vi "Actor Core.vi"(8 "error in":errorcluster, 11 "Freezer in":refnum<class "Freezer.lvclass">) -> (0 "error out":errorcluster, 3 "Actor out":refnum<class "Actor.lvclass">)   [LabVIEW 2015, in "cRIO-Carbondioxide.lvlib" / "CO2-Actor.lvlib" / "Freezer.lvclass"]
doc: "(<B>Filename</B>: Actor Framework.lvlib:Actor.lvclass:Actor Core.vi)\n\nReceives messages to the actor, reacts to them, and initiates any error handling that may shut the actor down.\n\nDescendant classes may override this VI to append parallel tasks for the actor to complete while it handles messages. Overrides use the Call Parent Method node."
uses:
  Freezer.lvclass
  <vilib>/ActorFramework/Actor/Actor.lvclass
  Freezer.lvclass/Freezer.ctl
  <vilib>/ActorFramework/Actor/Actor.lvclass/Actor.ctl
  <vilib>/ActorFramework/Message Enqueuer/Message Enqueuer.lvclass/Message Enqueuer.ctl
  Freezer Messages/Set Valve Msg/Set Valve Msg.lvclass/Set Valve Msg.ctl
  <vilib>/ActorFramework/Message Enqueuer/Enqueue.vi
  <vilib>/ActorFramework/Actor/Read Self Enqueuer.vi
  <vilib>/ActorFramework/Message Enqueuer/Init from Existing Queue.vi
  <vilib>/ActorFramework/Message Priority Queue/Priority Enqueue.vi
  CO2 Actor/CO2 Actor.lvclass
  Freezer Messages/Set Valve Msg/Set Valve Msg.lvclass
  <vilib>/ActorFramework/Message Enqueuer/Message Enqueuer.lvclass
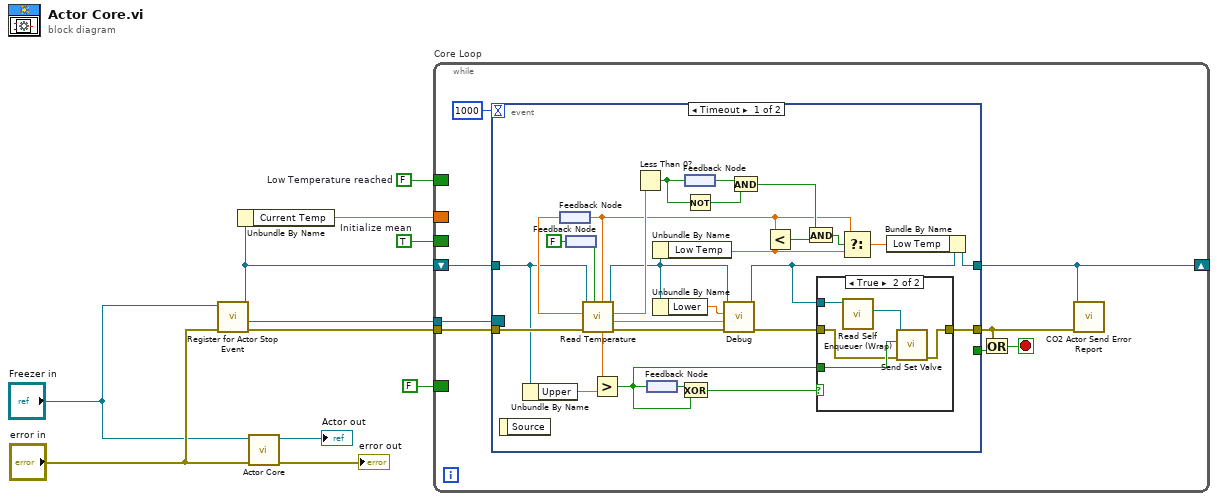
[diagram p0: block diagram]
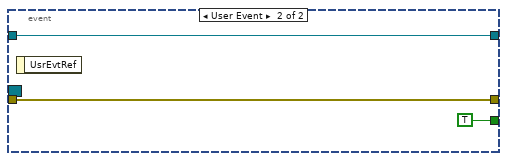
[diagram p3: hidden frame]
diagram:
  w9 = TRUE  # Initialize mean
  w10 = FALSE  # Low Temperature reached
  n1 = call "Register for Actor Stop Event.vi"("error in (no error)"="error in", "CO2 Actor in"="Freezer in") -> ("error out"=w4:errorcluster, "Event Registration Refnum"=w5:refnum<event-registration>, "CO2 Actor out"=w3:refnum<class "Freezer.lvclass">)  [unwired: 7 in]
  n2 = Unbundle By Name(w3) -> ("Current Temp"=w8:dbl)
  n3 = call-parent "Actor Core.vi"("error in"="error in", "CO2 Actor in"="Freezer in") -> ("error out"=→"error out":errorcluster, "Actor out"=→"Actor out":refnum<class "Actor.lvclass">)  [unwired: 8 in]
  n4 = while "Core Loop" {
    tunnel: w4 -> [w19]
    tunnel: w5 -> [w18]
    border: w10 -> [_]
    border: w9 -> [_]
    border: w8 -> [_]
    shift-right: [w12] -> _
    shift-left: w3 -> [w15]
    border: FALSE -> [_]
    stop <- w14 stop-if-true
    n5 = event shown="[0] Timeout" {
      selector: w18 -> [_ _]
      dyn-events: _ -> [_ _]
      timeout: 1000 -> [_ _]
      tunnel: w19 -> [w44 w54]
      tunnel: [_ TRUE] -> w17
      tunnel: w15 -> [w32 w55]
      tunnel: [w33 w54] -> w13
      tunnel: [w39 w55] -> w12
      event Timeout {
        n6 = event-data() -> ()  [unwired: 1 in, 1 out]
        n7 = Unbundle By Name(w32) -> ("Upper"=w31:dbl)
        n8 = feedback #1() -> (w42:dbl)
        n9 = feedback-in #2(FALSE) -> ()
        n10 = feedback #2() -> (w41:bool)
        n11 = call "Read Temperature.vi"("Initialize"=w41, "error in (no error)"=w44, "Current Temperature"=w42, "Freezer in"=w32) -> ("error out"=w25:errorcluster, "dT/dt"=w20:dbl, "dT/dt - Lower"=w40:dbl, "Freezer out"=w23:refnum<class "Freezer.lvclass">, "T - Low Temp"=w37:dbl, "T"=w26:dbl)  [unwired: 2 in]
        n12 = feedback-in #1(w26) -> ()
        n13 = Greater?(x=w37, y=w31) -> (0:w34:bool)
        n14 = Less Than 0?(x=w40) -> (x < 0?=w46:bool)
        n15 = feedback-in #3(w34) -> ()
        n16 = feedback #3() -> (w36:bool)
        n17 = Unbundle By Name(w23) -> ("Low Temp"=w27:dbl)
        n18 = Unbundle By Name(w23) -> ("Lower"=w21:dbl)
        n19 = Exclusive Or(1:w34, 2:w36) -> (0:w35:bool)
        n20 = feedback-in #4(w46) -> ()
        n21 = feedback #4() -> (w47:bool)
        n22 = Not(x=w46) -> (.not. x?=w45:bool)
        n23 = call "Debug.vi"("error in (no error)"=w25, "Numeric 2"=w20, "Numeric 1"=w21, "Freezer in"=w23) -> ("error out"=w24:errorcluster, "Freezer out"=w22:refnum<class "Freezer.lvclass">)  [unwired: 6 in]
        n24 = And(x=w47, y=w45) -> (x .and. y?=w29:bool)
        n25 = Less?(x=w26, y=w27) -> (x < y?=w28:bool)
        n26 = And(x=w29, y=w28) -> (x .and. y?=w30:bool)
        n27 = case shown="True" w35 {
          tunnel: w24 -> [w48 w50]
          tunnel: w22 -> [_ w51]
          tunnel: w34 -> [_ w52]
          tunnel: [w48 w53] -> w33
          frame False {
          }
          frame True {
            n28 = call "Read Self Enqueuer (Wrap).vi"("CO2 Actor in"=w51) -> ("Actor Framework:Message Enqueuer"=w49:refnum<class "Message Enqueuer.lvclass">)  [unwired: 9 in, 1 out]
            n29 = call "Send Set Valve.vi"("error in (no error)"=w50, "Open/Close"=w52, "Message Enqueuer"=w49) -> ("error out"=w53:errorcluster)  [unwired: 7 in, 1 out]
          }
        }
        n30 = Select(t=w26, s=w30, f=w27) -> (s? t:f=w38:dbl)
        n31 = Bundle By Name(cluster=w22, "Low Temp"=w38) -> (w39:refnum<class "Freezer.lvclass">)
      }
      event User Event {
        n32 = event-data() -> ()  [unwired: 1 in, 1 out]
      }
    }
    n33 = Or(x=w13, y=w17) -> (x .or. y?=w14:bool)
    n34 = call-dynamic "CO2 Actor Send Error Report.vi"("Error From Sender"=w13, "CO2 Actor in"=w12) -> ()  [unwired: 9 in, 1 out]
  }
